vi "Get Paths.vi"(8 "error in":errorcluster, 10 "Naming Data":refnum<class "Naming Data.lvclass">, 11 "Namer in":refnum<class "Namer.lvclass">) -> (0 "error out":errorcluster, 1 "Received Path":path, 2 "Approved Path":path, 3 "Namer out":refnum<class "Namer.lvclass">)   [LabVIEW 2020, in "Approval Tests.lvlib" / "Namer.lvclass"]
uses:
  Namer.lvclass
  Naming Data/Naming Data.lvclass
  Naming Data/Naming Data.lvclass/Naming Data.ctl
  Naming Data/Read Extension.vi
  Naming Data/Read Test Label.vi
  Naming Data/Read Test VI Name.vi
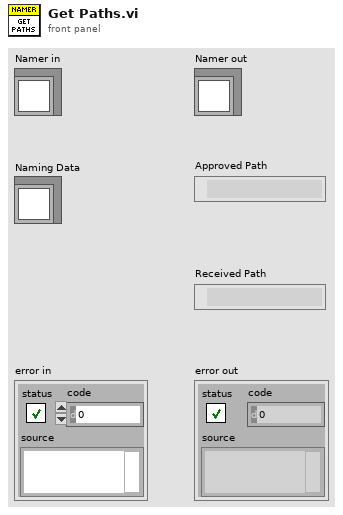
[diagram p1: front panel]
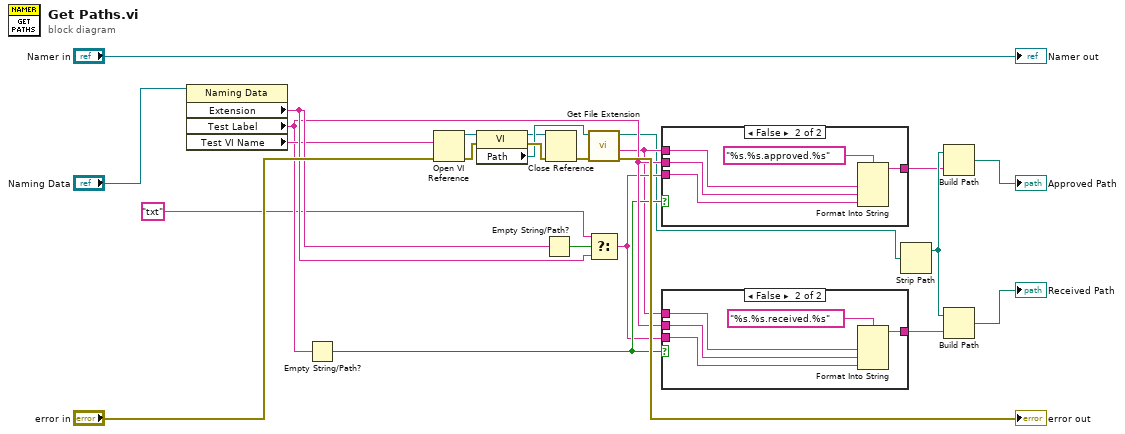
[diagram p0: block diagram]
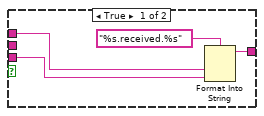
[diagram p2: hidden frame]
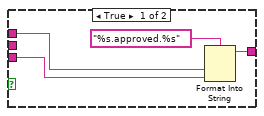
[diagram p3: hidden frame]
diagram:
  n1 = property class="Naming Data"(reference="Naming Data") -> ("Extension"=w15:string, "Test Label"=w13:string, "Test VI Name"=w14:string)  [unwired: 1 in, 2 out]
  n2 = Empty String/Path?(string/path=w13) -> (empty?=w12:bool)
  n3 = Open VI Reference(vi path=w14, error in (no error)="error in") -> (vi reference=w3:refnum<vi>, error out=w22:errorcluster)  [unwired: 4 in]
  n4 = property on="Property Node" class="VI"(reference=w3, error in=w22) -> (reference out=w1:refnum<vi>, error out=w21:errorcluster, "Path"=w2:path)
  n5 = Empty String/Path?(string/path=w15) -> (empty?=w9:bool)
  n6 = Close Reference(reference=w1, error in (no error)=w21) -> (error out=w20:errorcluster)
  n7 = call <vilib>:"Get File Extension.vi"("error in (no error)"=w20, "file"=w2) -> ("error out"=→"error out":errorcluster, "filename without extension"=w8:string, "dup file"=w5:path)  [unwired: 5 in, 2 out]
  n8 = Select(t="txt", s=w9, f=w15) -> (s? t:f=w10:string)
  n9 = case shown="False" w12 {
    tunnel: [w28 w32] -> w4
    tunnel: w8 -> [w27 w31]
    tunnel: w10 -> [w25 w30]
    tunnel: w13 -> [_ w29]
    frame True {
      n10 = Format Into String(format string="%s.approved.%s", w27, w25) -> (resulting string=w28:string)  [unwired: 2 in, 1 out]
    }
    frame False {
      n11 = Format Into String(format string="%s.%s.approved.%s", w31, w29, w30) -> (resulting string=w32:string)  [unwired: 2 in, 1 out]
    }
  }
  n12 = case shown="False" w12 {
    tunnel: [w36 w41] -> w6
    tunnel: w8 -> [w35 w40]
    tunnel: w10 -> [w34 w38]
    tunnel: w13 -> [_ w39]
    frame True {
      n13 = Format Into String(format string="%s.received.%s", w35, w34) -> (resulting string=w36:string)  [unwired: 2 in, 1 out]
    }
    frame False {
      n14 = Format Into String(format string="%s.%s.received.%s", w40, w39, w38) -> (resulting string=w41:string)  [unwired: 2 in, 1 out]
    }
  }
  n15 = Strip Path(path=w5) -> (stripped path=w7:path)  [unwired: 1 out]
  n16 = Build Path(base path=w7, name or relative path=w4) -> (appended path=→"Approved Path":path)
  n17 = Build Path(base path=w7, name or relative path=w6) -> (appended path=→"Received Path":path)
  "Namer out" <- "Namer in"
